vi "Increase Counter.vi"(8 "error in (no error)":errorcluster, 11 "Packet in":refnum<class "Packet.lvclass">) -> (0 "error out":errorcluster, 3 "Packet out":refnum<class "Packet.lvclass">)   [LabVIEW 2020, in "Communication Classes.lvlib" / "Packet.lvclass"]
uses:
  Packet.lvclass
  Packet.lvclass/Packet.ctl
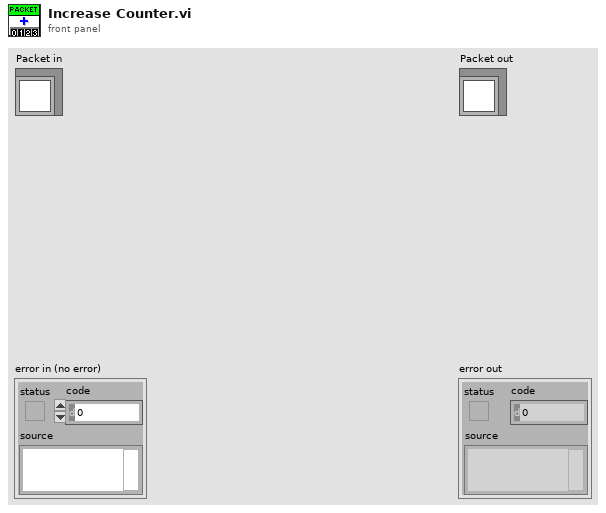
[diagram p1: front panel]
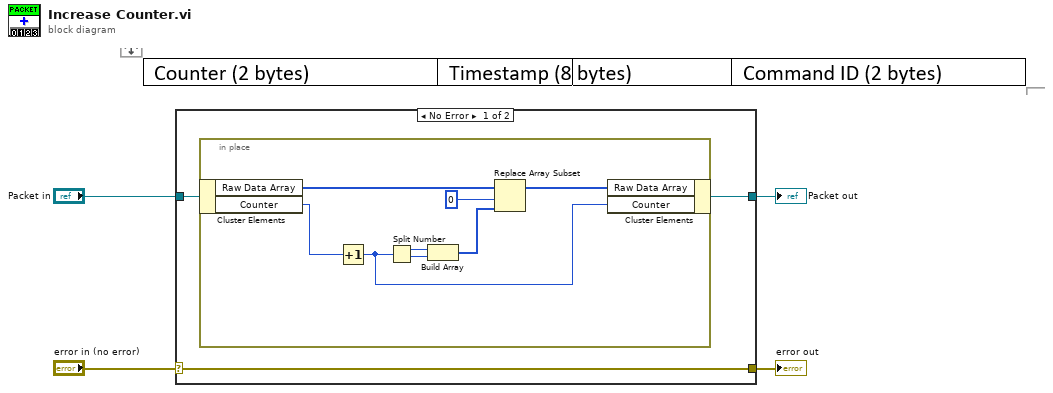
[diagram p0: block diagram]
diagram:
  n1 = case shown="No Error" "error in (no error)" {
    selector: "error in (no error)" -> [w7 w16]
    tunnel: [w7 w16] -> w3
    tunnel: [w5 w17] -> w1
    tunnel: "Packet in" -> [w6 w17]
    frame No Error {
      n2 = in-place {
        n3 = in-place-cluster #1(w6) -> ("Raw Data Array"=w15:u8[], "Counter"=w9:u16)
        n4 = Increment(x=w9) -> (x+1=w8:u16)
        n5 = Split Number(x=w8) -> (hi(x)=w13:u8, lo(x)=w12:u8)
        n6 = Build Array(w13, w12) -> (w11:u8[])
        n7 = Replace Array Subset "Replace Array Subset"(array=w15, new element=w11, index=0) -> (w14:u8[])
        n8 = in-place-cluster #1("Raw Data Array"=w14, "Counter"=w8) -> (w5:refnum<class "Packet.lvclass">)
      }
    }
    frame Error {
    }
  }
  "error out" <- w3
  "Packet out" <- w1
